vi "List DQMH.vi"() -> ()   [LabVIEW 2020]
uses:
  <vilib>/National Instruments/Tree Map/Tree Map Data.ctl
  Scripting/Event types--enum.ctl
  <vilib>/National Instruments/Tree Map/API/List Roots.vi
  <vilib>/National Instruments/Tree Map/Utility/Into Tree Control Items.vi
  Scripting/DQMH_API.lvlib
  <vilib>/National Instruments/Tree Map/Tree Map.lvlib
  <vilib>/ProgressBar/Progress Bar Dialog.lvclass
panel:
  out "Module":string
  in  "Refresh":bool
  in  "Lists":string(tree) caption="Tree 2"
  in  "Module ID":i32 caption="Numeric"
  out "Running?":bool
  in  "Open API Tester":bool
  in  "Run Request VI":bool
  in  "Show Block Diagram":bool
  in  "Hide Front Panel":bool
  in  "Show Front Panel":bool
  in  "Stop All":bool
  in  "Stop Module":bool
  out "Connector pane":picture
  out "Vi Documentation":string
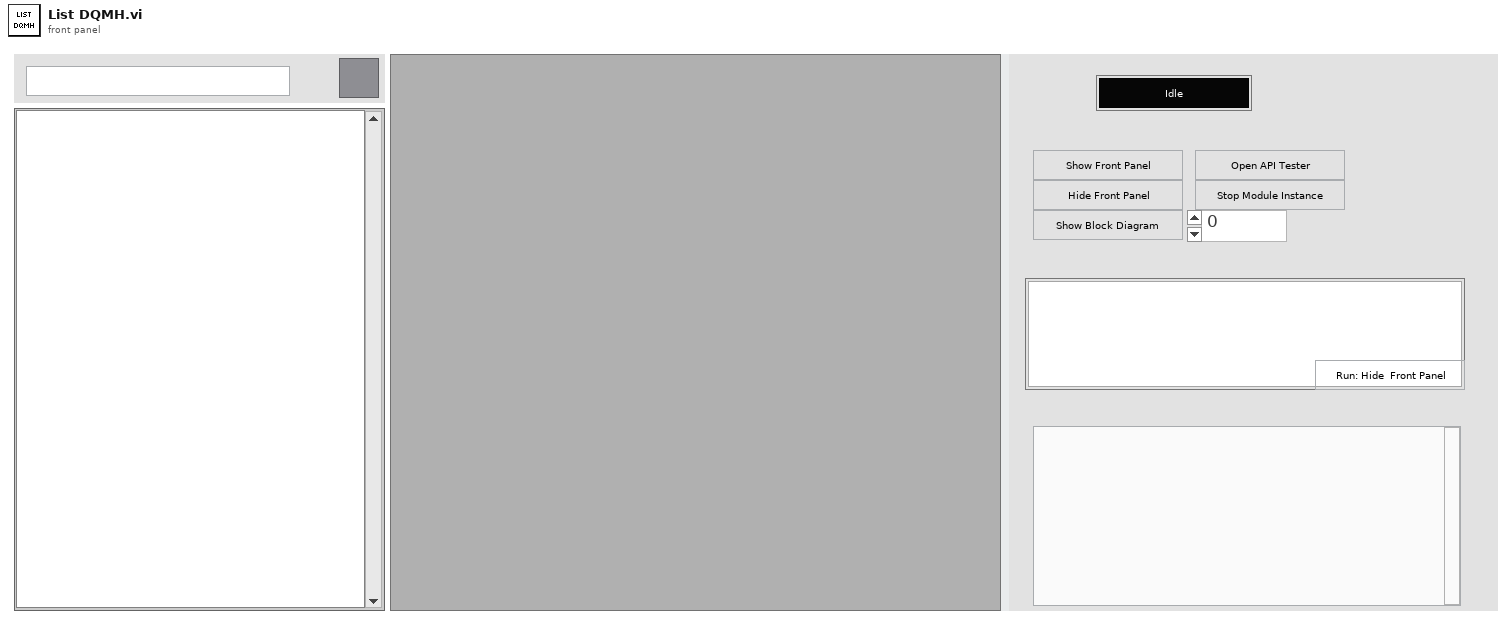
[diagram p1: front panel]
types:
  T1 = enum32{"Invalid", "Standard", "Closed", "Hidden", "Minimized", "Maximized"}
  T2 = enum32{"invalid app kind", "Development System", "Run Time System", "Student Edition", "Embedded LabVIEW", "Evaluation", "Custom"}
  T3 = typedef "Tree Map.lvlib/Tree Map Data.ctl" = map{string, cluster{"Child Paths Set":set{string}, "Name":string, "Data":string, "Attributes":map{string, string}}}
  T4 = cluster{"Core":cluster{"Current VI Reference":refnum<vi>, "Close Panel on Exit?":bool}, "Lists ref":refnum<vi>, "Sub Panel":refnum<vi>, "Tree Map":T3, "References Map":map{string, refnum<vi>}, "vi Ref":refnum<vi>, "Module ID":i32}
  T5 = cluster{"Child Paths Set":set{string}, "Name":string, "Data":string, "Attributes":map{string, string}}
  T6 = cluster{"Current VI Reference":refnum<vi>, "Close Panel on Exit?":bool}
  T7 = typedef "DQMH_API.lvlib/Event types--enum.ctl" = enum16{"Request", "Request and Wait for Reply", "Broadcast"}
  T8 = cluster{"Left Cell String":string, "Child Text":string[], "Child Tag":string, "Item Indent":i32, "Child Only?":bool, "Glyph Index":i32}[]
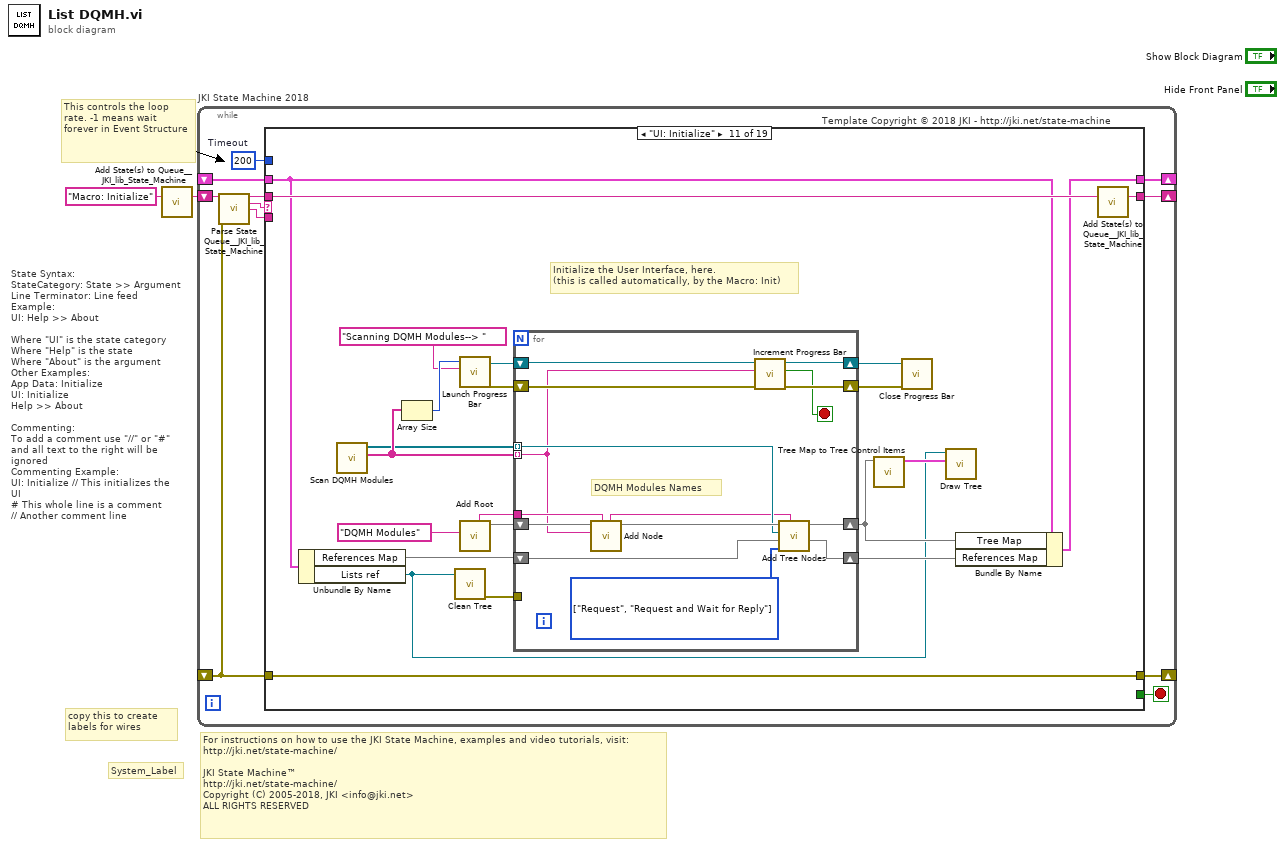
[diagram p0: block diagram]
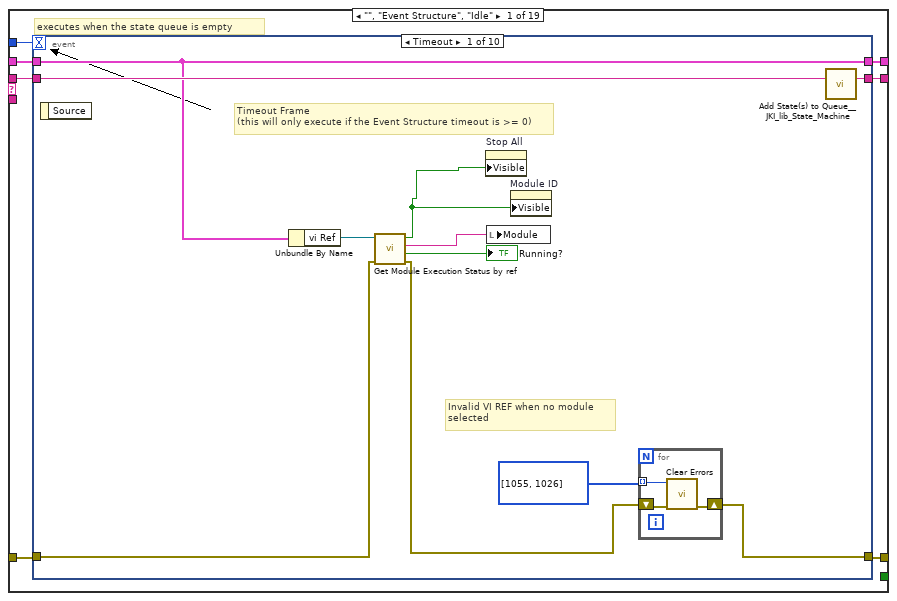
[diagram p2: hidden frame]
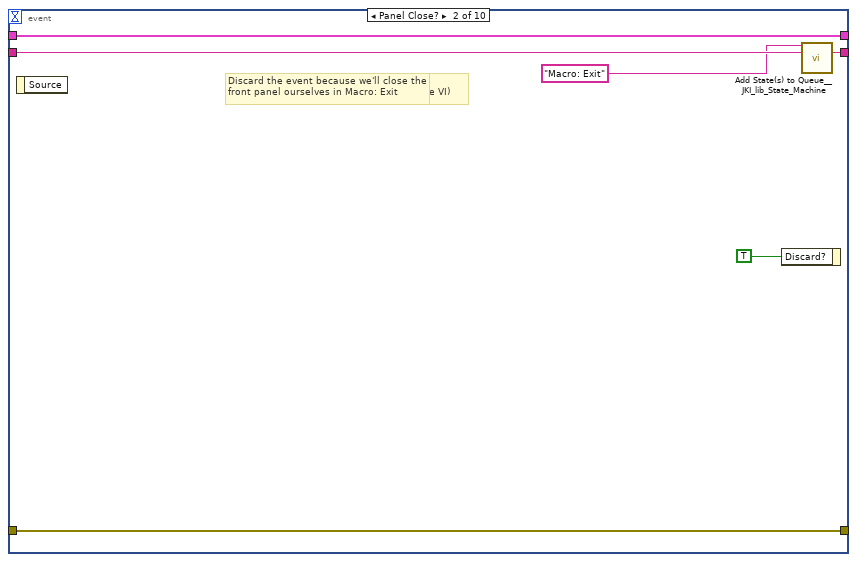
[diagram p3: hidden frame]
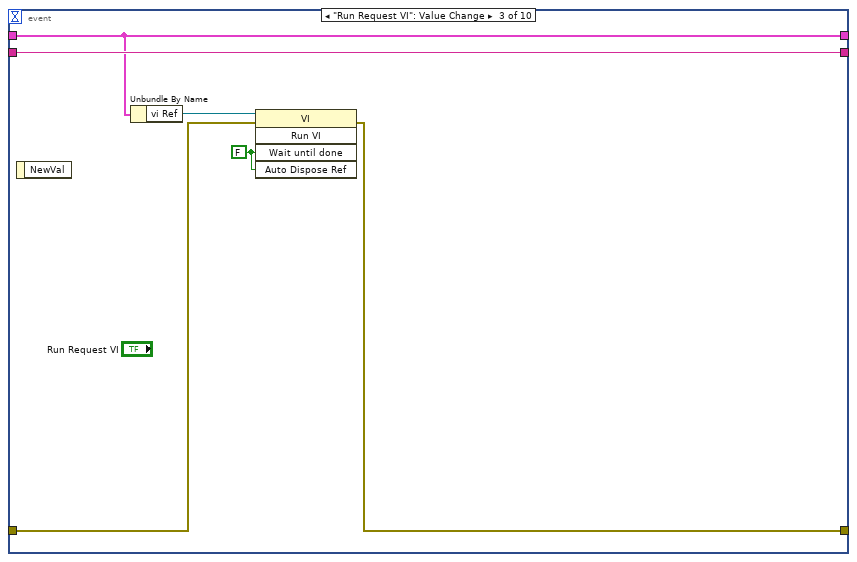
[diagram p4: hidden frame]
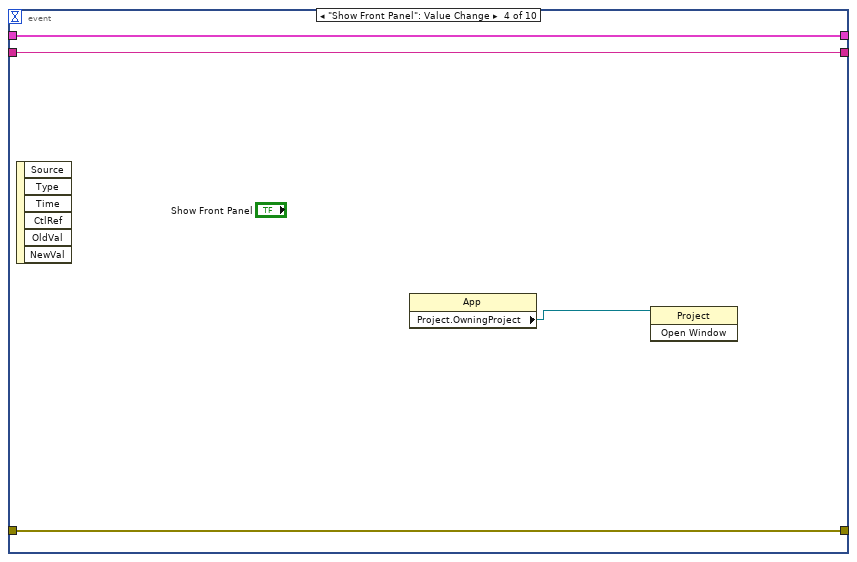
[diagram p5: hidden frame]
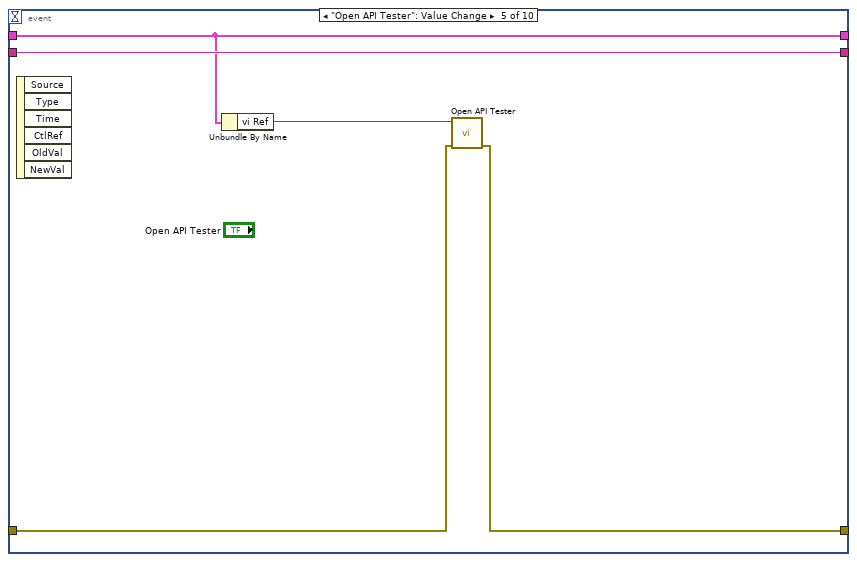
[diagram p6: hidden frame]
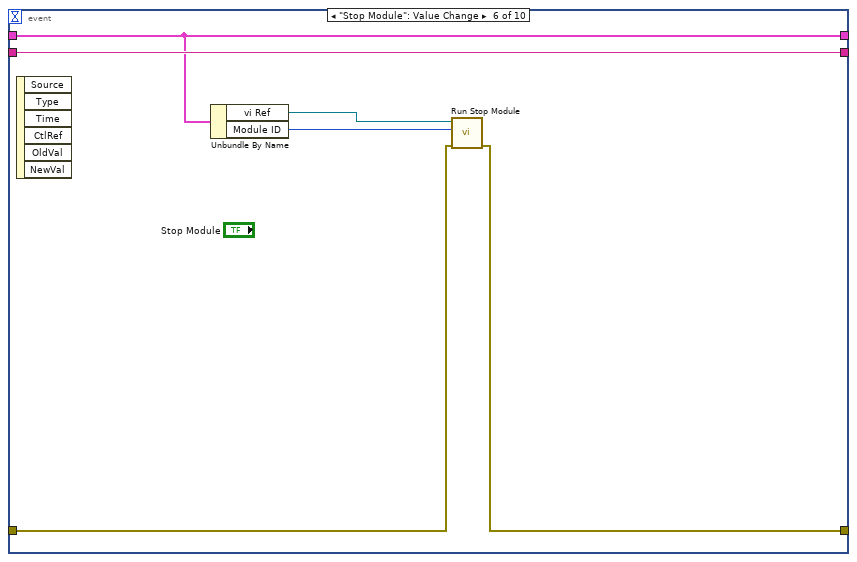
[diagram p7: hidden frame]
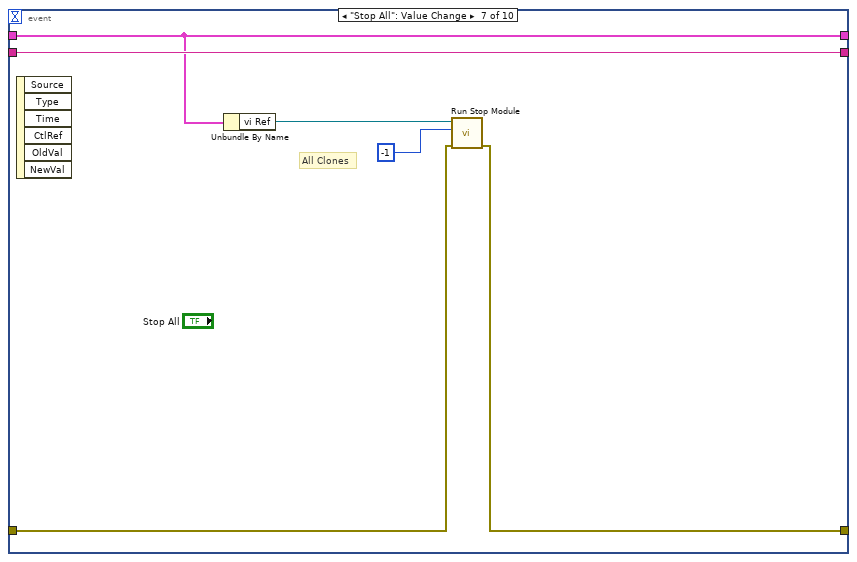
[diagram p8: hidden frame]
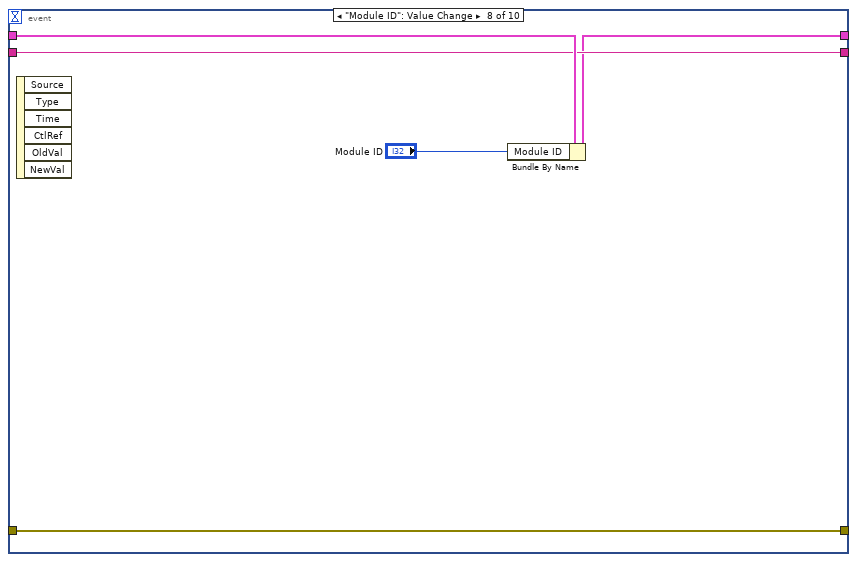
[diagram p9: hidden frame]
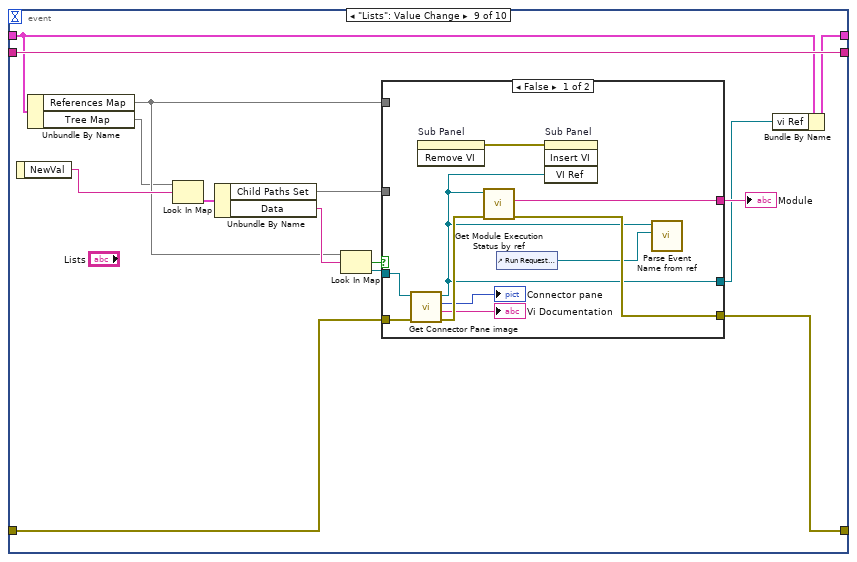
[diagram p10: hidden frame]
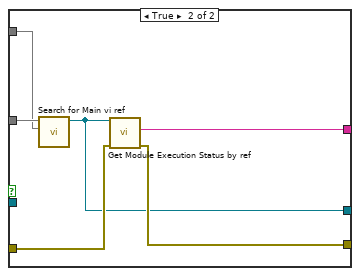
[diagram p11: hidden frame]
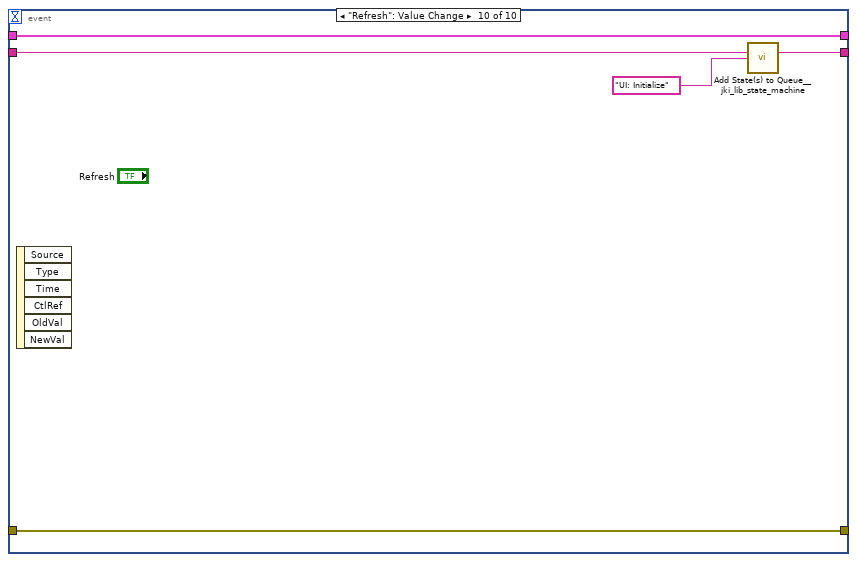
[diagram p12: hidden frame]
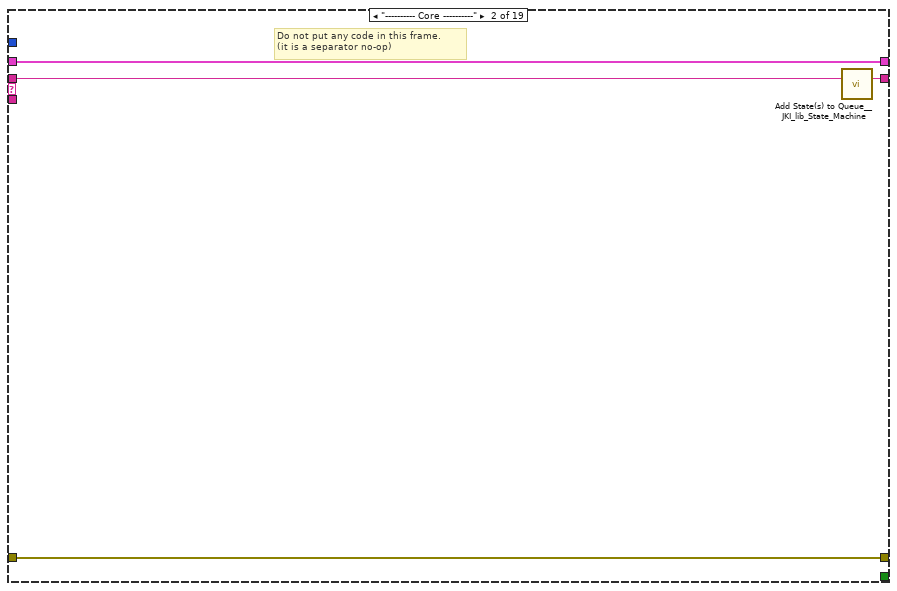
[diagram p13: hidden frame]
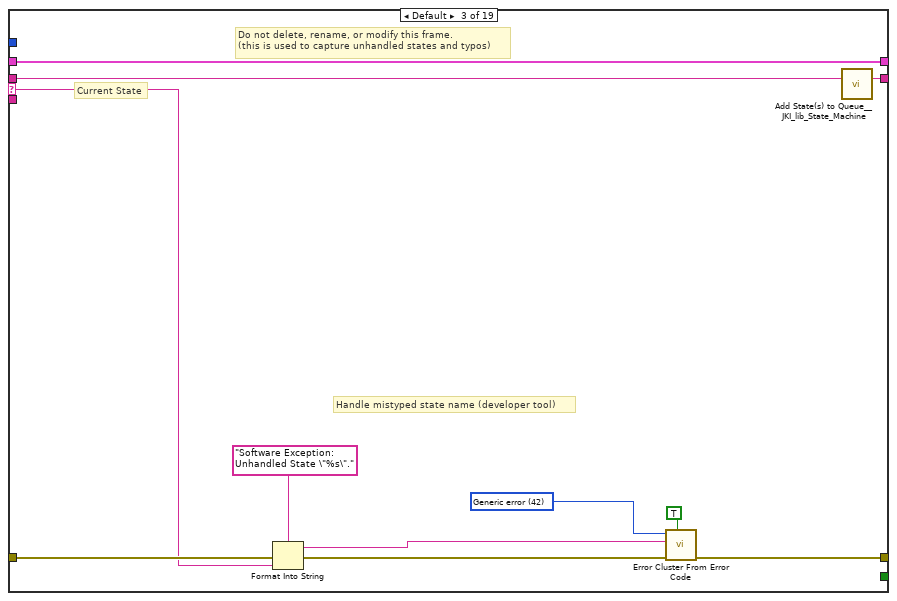
[diagram p14: hidden frame]
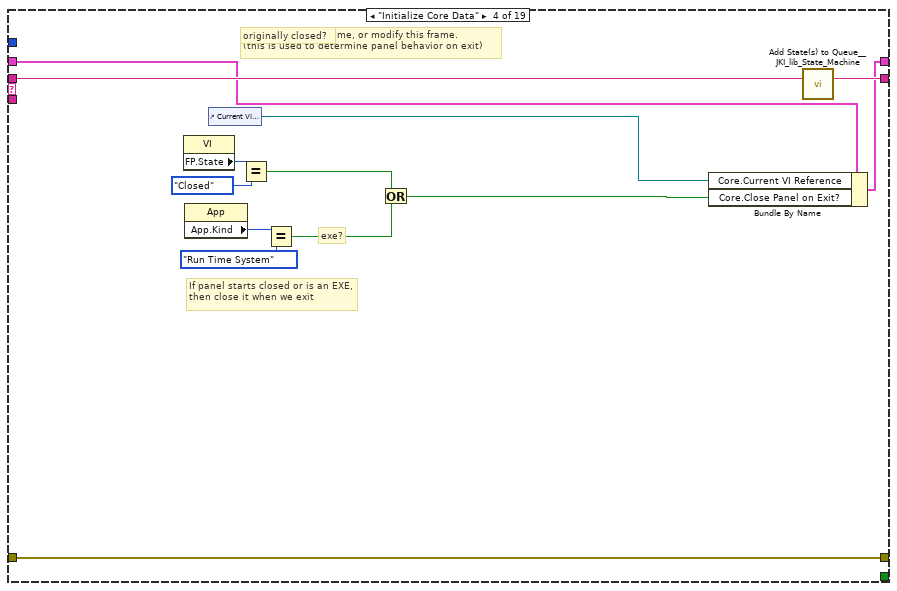
[diagram p15: hidden frame]
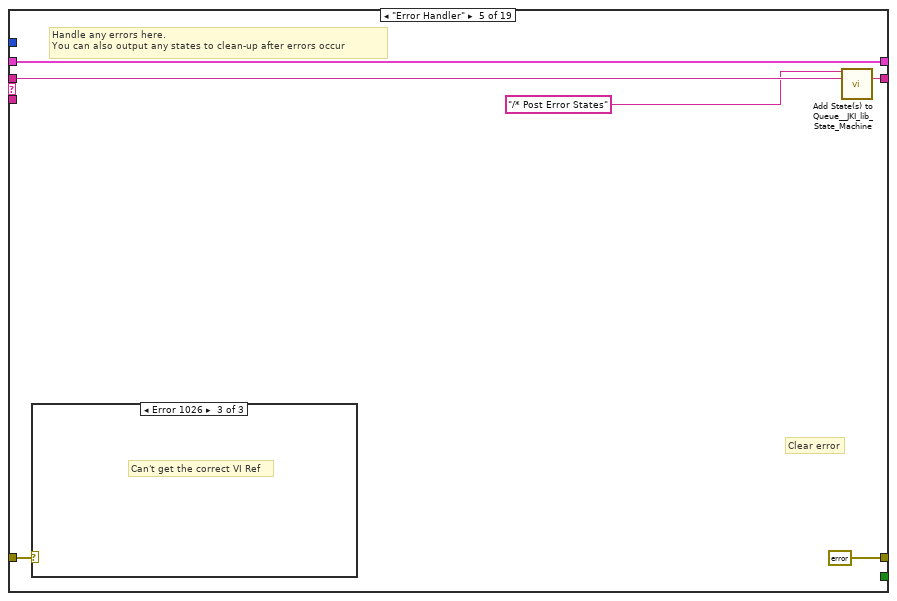
[diagram p16: hidden frame]
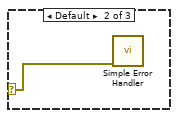
[diagram p18: hidden frame]
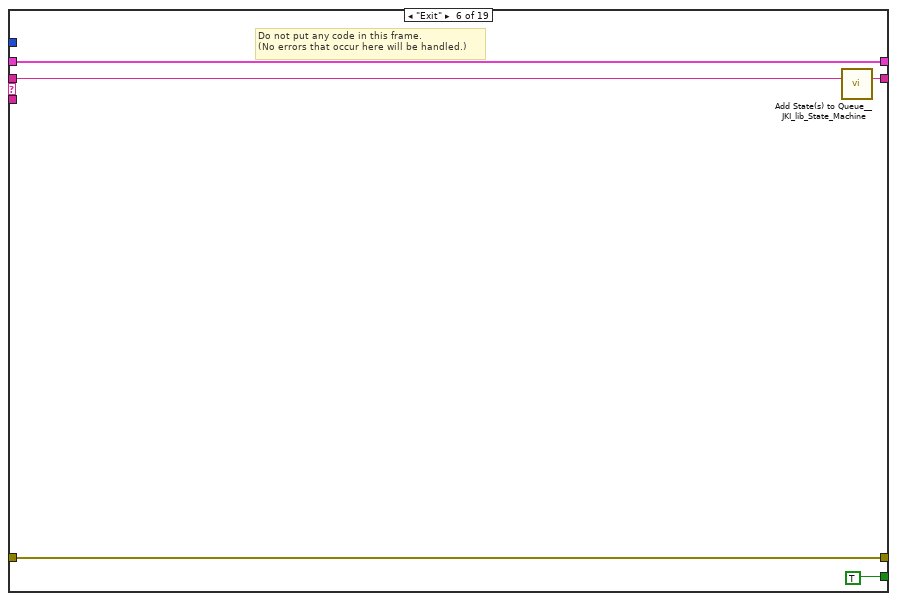
[diagram p19: hidden frame]
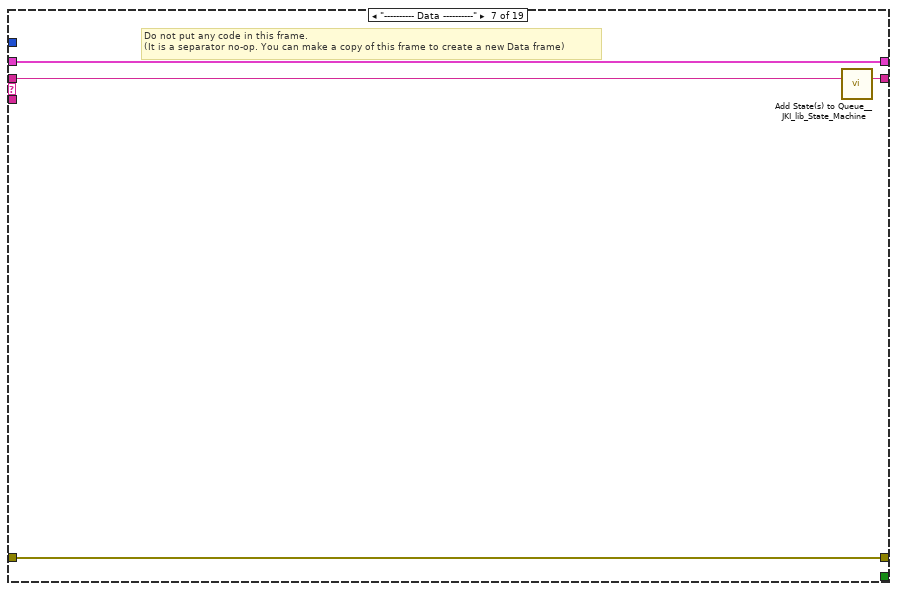
[diagram p20: hidden frame]
diagram:
  # "For instructions on how to use the JKI State Machine, examples and video tutorials, visit:\nhttp://jki.net/state-machine/\n\nJKI State Machine™\nhttp://jki.net/state-machine/\nCopyright (C) 2005-2018, JKI <info@jki.net>\nALL RIGHTS RESERVED"
  # "State Syntax:\nStateCategory: State >> Argument\nLine Terminator: Line feed\nExample:\nUI: Help >> About\n\nWhere \"UI\" is the state category\nWhere \"Help\" is the state\nWhere \"About\" is the argument\nOther Examples:\nApp Data: Initialize\nUI: Initialize\nHelp >> About\n\nCommenting:\nTo add a comment use \"//\" or \"#\" and all text to the right will be ignored\nCommenting Example:\nUI: Initialize // This initializes the UI\n# This whole line is a comment\n// Another comment line"
  # "copy this to create labels for wires"
  # "This controls the loop rate. -1 means wait forever in Event Structure"
  # "System_Label"
  n1 = call <vilib>:"Add State(s) to Queue__JKI_lib_State_Machine.vi"("State(s) in (\"\")"="Macro: Initialize") -> ("States Out"=w2:string)  [unwired: 14 in]
  n2 = while "JKI State Machine 2018" {
    shift-right: [w5] -> _
    shift-left: _ -> [w4]
    shift-right: [w13] -> _
    shift-left: _ -> [w12]
    shift-right: [w7] -> _
    shift-left: w2 -> [w8]
    stop <- w6 stop-if-true
    w3 = 200  # Timeout
    # "Template Copyright © 2018 JKI - http://jki.net/state-machine"
    n3 = call <vilib>:"Parse State Queue__JKI_lib_State_Machine.vi"("State Queue"=w8, "Error In (no error)"=w12) -> ("Remaining States"=w10:string, "Current State"=w11:string, "Arguments"=w9:string)  [unwired: 11 in]
    n4 = case shown="\"UI: Initialize\"" w11 {
      selector: w11 -> [_ _ w113 _ _ _ _ _ _ _ _ _ _ _ _ _ _ _ _]
      tunnel: w10 -> [w18 w111 w117 w135 w140 w147 w151 w162 w170 w179 w198 w221 w232 w297 w302 w312 w316 w320 w324]
      tunnel: w9 -> [_ _ _ _ _ _ _ _ _ _ _ w218 w229 _ _ _ _ _ _]
      tunnel: w4 -> [w16 w109 w115 w124 w138 w144 w149 _ w165 w177 w183 w219 w228 w295 w300 w305 w314 w318 w322]
      tunnel: [w20 w112 w122 w136 errorcluster {"status"=FALSE, "code"=0, "source"=""} ("error out") w148 w152 w163 w174 w180 w202 w222 w233 w298 w303 w313 w317 w321 w325] -> w13
      tunnel: w12 -> [w19 w112 w121 w136 w141 w148 w152 w163 w176 w180 w202 w223 w234 w298 w303 w313 w317 w321 w325]
      tunnel: [w17 w110 w116 w134 w139 w146 w150 w161 w169 w178 w197 w220 w231 w296 w301 w311 w315 w319 w323] -> w7
      tunnel: [_ _ _ _ _ TRUE _ _ _ _ _ _ _ _ _ _ _ _ _] -> w6
      tunnel: [w14 w109 w115 w125 w138 w144 w149 w154 w165 w177 w184 w219 w228 w295 w300 w305 w314 w318 w322] -> w5
      tunnel: w3 -> [w15 _ _ _ _ _ _ _ _ _ _ _ _ _ _ _ _ _ _]
      frame "", "Event Structure", "Idle" {
        # "executes when the state queue is empty"
        n5 = event shown="[0] Timeout" {
          selector: _ -> [_ _ _ _ _ _ _ _ _ _]
          dyn-events: _ -> [_ _ _ _ _ _ _ _ _ _]
          timeout: w15 -> [_ _ _ _ _ _ _ _ _ _]
          tunnel: w18 -> [w28 w39 w44 w49 w53 w59 w65 w70 w79 w105]
          tunnel: [w27 w38 w44 w49 w53 w59 w65 w70 w79 w106] -> w17
          tunnel: w16 -> [w26 w35 w42 w48 w52 w58 w64 w71 w75 w107]
          tunnel: [w29 w40 w45 w50 w55 w61 w67 w72 w86 w108] -> w20
          tunnel: w19 -> [w31 w40 w46 w50 w54 w60 w66 w72 w87 w108]
          tunnel: [w26 w35 w42 w48 w52 w58 w64 w69 w78 w107] -> w14
          event Timeout {
            # "Invalid VI REF when no module \nselected"
            # "Timeout Frame\n(this will only execute if the Event Structure timeout is >= 0)"
            n6 = event-data() -> ()  [unwired: 1 in, 1 out]
            n7 = Unbundle By Name(w26) -> ("vi Ref"=w25:refnum<vi>)
            n8 = call "Get Module Execution Status by ref.vi"("error in"=w31, "Vi Ref"=w25) -> ("error out"=w30:errorcluster, "Running?"=→"Running?":bool, "Module Name"=w24:string, "Is Cloneable"=w21:bool)  [unwired: 6 in]
            n9 = property on="Stop All" class="Bool"("Visible"=w21) -> ()  [unwired: 2 in, 2 out]
            n10 = local write "Module"(w24) -> ()
            n11 = property on="Module ID" class="DigNum (strict)"("Visible"=w21) -> ()  [unwired: 2 in, 2 out]
            n12 = for {
              tunnel: i32[] [1055, 1026] ("specific error code to clear (0: all)") -> [w32] mode=indexing
              shift-right: [w33] -> w29
              shift-left: w30 -> [w34]
              n13 = call <vilib>:"Clear Errors.vi"("error in (no error)"=w34, "specific error code to clear (0: all)"=w32) -> ("error out"=w33:errorcluster)  [unwired: 4 in, 1 out]
            }
            n14 = call <vilib>:"Add State(s) to Queue__JKI_lib_State_Machine.vi"("State(s) in (\"\")"=w28) -> ("States Out"=w27:string)  [unwired: 14 in]
          }
          event Panel Close? {
            # "Discard the event because we'll close the front panel ourselves in Macro: Exit"
            # "Close Panel button (pressed) Event\n(this executes Macro: Exit to terminate the VI)"
            n15 = event-data() -> ()  [unwired: 1 in, 1 out]
            n16 = event-data("Discard?"=TRUE) -> ()  [unwired: 1 in, 1 out]
            n17 = call <vilib>:"Add State(s) to Queue__JKI_lib_State_Machine.vi"("State(s) in Front (\"\")"="Macro: Exit", "State(s) in (\"\")"=w39) -> ("States Out"=w38:string)  [unwired: 13 in]
          }
          event "Run Request VI": Value Change {
            w43 = FALSE ("Wait Until Done")
            n18 = event-data() -> ()  [unwired: 1 in, 1 out]
            n19 = Unbundle By Name(w42) -> ("vi Ref"=w41:refnum<vi>)
            n20 = invoke class="VI" method="Run VI"(reference=w41, error in=w46, "Wait until done"=w43, "Auto Dispose Ref"=w43) -> (error out=w45:errorcluster)  [unwired: 1 in, 4 out]
          }
          event "Show Front Panel": Value Change {
            n21 = event-data() -> ()  [unwired: 1 in, 6 out]
            n22 = property class="App"() -> ("Project.OwningProject"=w47:refnum<vi>)  [unwired: 2 in, 2 out]
            n23 = invoke class="Project" method="Open Window"(reference=w47) -> ()  [unwired: 2 in, 3 out]
          }
          event "Open API Tester": Value Change {
            n24 = event-data() -> ()  [unwired: 1 in, 6 out]
            n25 = Unbundle By Name(w52) -> ("vi Ref"=w51:refnum<vi>)
            n26 = call "Open API Tester.vi"("error in"=w54, "Event vi Ref"=w51) -> ("error out"=w55:errorcluster)  [unwired: 9 in]
          }
          event "Stop Module": Value Change {
            n27 = event-data() -> ()  [unwired: 1 in, 6 out]
            n28 = Unbundle By Name(w58) -> ("vi Ref"=w57:refnum<vi>, "Module ID"=w56:i32)
            n29 = call "Run Stop Module.vi"("error in"=w60, "Module ID"=w56, "Event vi Ref"=w57) -> ("error out"=w61:errorcluster)  [unwired: 8 in]
          }
          event "Stop All": Value Change {
            # "All Clones"
            n30 = event-data() -> ()  [unwired: 1 in, 6 out]
            n31 = Unbundle By Name(w64) -> ("vi Ref"=w63:refnum<vi>)
            n32 = call "Run Stop Module.vi"("error in"=w66, "Module ID"=-1, "Event vi Ref"=w63) -> ("error out"=w67:errorcluster)  [unwired: 8 in]
          }
          event "Module ID": Value Change {
            n33 = event-data() -> ()  [unwired: 1 in, 6 out]
            n34 = Bundle By Name(cluster=w71, "Module ID"="Module ID") -> (w69:T4)
          }
          event "Lists": Value Change {
            n35 = event-data() -> ("NewVal"=w84:string)  [unwired: 1 in]
            n36 = Unbundle By Name(w75) -> ("References Map"=w74:map{string, refnum<vi>}, "Tree Map"=w73:T3)
            n37 = Look In Map(map=w73, key=w84) -> (value=w85:T5)  [unwired: 1 in, 1 out]
            n38 = Unbundle By Name(w85) -> ("Child Paths Set"=w81:set{string}, "Data"=w83:string)
            n39 = Look In Map(map=w74, key=w83) -> (key not found?=w82:bool, value=w76:refnum<vi>)  [unwired: 1 in]
            n40 = case shown="False" w82 {
              tunnel: [w88 w99] -> w77
              tunnel: [w92 w100] -> w80
              tunnel: w74 -> [_ w98]
              tunnel: w81 -> [_ w101]
              tunnel: w76 -> [w91 _]
              tunnel: w87 -> [w96 w103]
              tunnel: [w94 w102] -> w86
              frame False {
                n41 = call "Get Connector Pane image.vi"("error in"=w96, "VI in"=w91) -> ("error out"=w95:errorcluster, "VI Description"=→"Vi Documentation":string, "Connector pane Image"=→"Connector pane":picture, "Vi out"=w88:refnum<vi>)  [unwired: 6 in]
                n42 = invoke on="Sub Panel" class="SubPnl" method="Remove VI"() -> (error out=w97:errorcluster)  [unwired: 3 in, 2 out]
                n43 = call "Get Module Execution Status by ref.vi"("error in"=w95, "Vi Ref"=w88) -> ("error out"=w94:errorcluster, "Module Name"=w92:string)  [unwired: 6 in, 2 out]
                n44 = control-ref of="Run Request VI"() -> (w89:refnum<vi>)
                n45 = invoke on="Sub Panel" class="SubPnl" method="Insert VI"(error in=w97, "VI Ref"=w88) -> ()  [unwired: 2 in, 4 out]
                n46 = call "Parse Event Name from ref.vi"("Boolean Run Request VI"=w89, "VI in"=w88) -> ()  [unwired: 10 in]
              }
              frame True {
                n47 = call "Search for Main vi ref.vi"("map"=w98, "Child Paths Set"=w101) -> ("Main vi Ref"=w99:refnum<vi>)  [unwired: 9 in]
                n48 = call "Get Module Execution Status by ref.vi"("error in"=w103, "Vi Ref"=w99) -> ("error out"=w102:errorcluster, "Module Name"=w100:string)  [unwired: 6 in, 2 out]
              }
            }
            "Module" <- w80
            n49 = Bundle By Name(cluster=w75, "vi Ref"=w77) -> (w78:T4)
          }
          event "Refresh": Value Change {
            n50 = event-data() -> ()  [unwired: 1 in, 6 out]
            n51 = call <vilib>:"Add State(s) to Queue__jki_lib_state_machine.vi"("State(s) in (\"\")"=w105, "State(s) at Back (\"\")"="UI: Initialize" ("State(s) at Back (\"\")")) -> ("States Out"=w106:string)  [unwired: 13 in]
          }
        }
      }
      frame "---------- Core ----------" {
        # "Do not put any code in this frame.\n(it is a separator no-op)"
        n52 = call <vilib>:"Add State(s) to Queue__JKI_lib_State_Machine.vi"("State(s) in (\"\")"=w111) -> ("States Out"=w110:string)  [unwired: 14 in]
      }
      frame Default {
        w119 = 42 items=["No error", "Argument error", "Memory is full", "Out of zone", "End of file", "File already open", "Generic file I/O error", "File not found", "File permission error", "Disk is full", "Duplicate path", "Too many files open", "System feature not enabled", "Resource file not found", "Cannot add resource", "Resource not found", "Image not found", "Image memory error", "Pen does not exist", "Config type invalid", "Config token not found", "Config parse error", "Config memory error", "Bad external code format", "Bad external code offset", "External code not present", "Null window", "Destroy window error", "Null menu", "Print aborted", "Bad print record", "Print driver error", "Windows error during printing", "Memory error during printing", "Print dialog error", "Generic print error", "Invalid device refnum", "Device not found", "Device parameter error", "Device unit error", "Cannot open device", "Device call aborted", "Generic error", "Cancelled by user", "Object ID too low", "Object ID too high", "Object not in heap", "Unknown heap", "Unknown object (invalid DefProc)", "Unknown object (DefProc not in table)", "Message out of range", "Invalid (null) method", "Unknown message", "Manager call not supported", "Bad address", "Network operation in progress", "Network operation timed out", "Connection is busy", "Network attribute not supported", "Network error", "Address in use", "System out of memory", "Connection aborted", "Connection refused", "Not connected", "Already connected", "Connection closed", "Initialization error (interapplication manager)", "Bad occurrence", "Wait on unbound occurrence handler", "Occurrence queue overflow", "Datalog type conflict", "Unused", "Unrecognized type (interapplication manager)", "Memory corrupt", "Failed to make temporary DLL", "Old CIN version", "Drag socket not found", "Failed to load drop-object", "Failed to register OLE object", "Failed to release OLE object", "Format specifier type mismatch", "Unknown format specifier", "Too few format specifiers", "Too many format specifiers", "Scan failed", "Newer CIN version", "Error converting to variant", "Runtime menu error", "Password tampered", "Variant attribute not found", "Incompatible variant data type", "Event data is not available", "Event Store is not present", "Occurrence is not found", "Event Queue is not created", "Event info is not available", "Refnum passed is NULL", "Error retrieving Class GUID", "Error retrieving CoClass GUID", "Error retrieving TypeLib GUID.", "Bad built application magic bytes.", "Specific driver is different from the specific driver associated with the Logical Name.", "There is no session opened to the class driver.", "Max Error", "MAX - Error with config objects", "MAX - Error loading configuration", "MAX - Group not supported"]
        # "Current State"
        # "Do not delete, rename, or modify this frame.\n(this is used to capture unhandled states and typos)"
        # "Handle mistyped state name (developer tool)"
        n53 = Format Into String(format string="Software Exception: Unhandled State \"%s\"." ("message"), error in=w121, w113) -> (resulting string=w118:string, error out=w123:errorcluster)  [unwired: 1 in]
        n54 = call <vilib>:"Error Cluster From Error Code.vi"("show call chain? (False)"=TRUE, "error in (no error)"=w123, "error message (\"\")"=w118, "error code (0)"=w119) -> ("error out"=w122:errorcluster)  [unwired: 5 in]
        n55 = call <vilib>:"Add State(s) to Queue__JKI_lib_State_Machine.vi"("State(s) in (\"\")"=w117) -> ("States Out"=w116:string)  [unwired: 14 in]
      }
      frame "Initialize Core Data" {
        # "Do not delete, rename, or modify this frame.\n(this is used to determine panel behavior on exit)"
        # "originally closed?"
        # "exe?"
        # "If panel starts closed or is an EXE, then close it when we exit"
        n56 = property class="VI"() -> ("FP.State"=w128:T1)  [unwired: 2 in, 2 out]
        n57 = property class="App"() -> ("App.Kind"=w133:T2)  [unwired: 2 in, 2 out]
        n58 = control-ref of="Current VI Reference"() -> (w129:refnum<vi>)
        n59 = Equal?(x=w128, y=T1."Closed" ("Front Panel Window:State")) -> (x = y?=w126:bool)
        n60 = Equal?(x=w133, y=T2."Run Time System" ("Application:Kind")) -> (x = y?=w131:bool)
        n61 = Or(x=w126, y=w131) -> (x .or. y?=w130:bool)
        n62 = Bundle By Name(cluster=w124, "Core.Current VI Reference"=w129, "Core.Close Panel on Exit?"=w130) -> (w125:T4)
        n63 = call <vilib>:"Add State(s) to Queue__JKI_lib_State_Machine.vi"("State(s) in (\"\")"=w135) -> ("States Out"=w134:string)  [unwired: 14 in]
      }
      frame "Error Handler" {
        # "Handle any errors here.\nYou can also output any states to clean-up after errors occur"
        # "Clear error"
        n64 = case shown="Error 1026" w141 {
          selector: w141 -> [_ w143 _]
          frame No Error {
          }
          frame Default {
            n65 = call <vilib>:"Simple Error Handler.vi"("error in (no error)"=w143) -> ()  [unwired: 4 in, 5 out]
          }
          frame Error {
            # "Can't get the correct VI Ref"
          }
        }
        n66 = call <vilib>:"Add State(s) to Queue__JKI_lib_State_Machine.vi"("State(s) in Front (\"\")"="/* Post Error States", "State(s) in (\"\")"=w140) -> ("States Out"=w139:string)  [unwired: 13 in]
      }
      frame "Exit" {
        # "Do not put any code in this frame.\n(No errors that occur here will be handled.)"
        n67 = call <vilib>:"Add State(s) to Queue__JKI_lib_State_Machine.vi"("State(s) in (\"\")"=w147) -> ("States Out"=w146:string)  [unwired: 14 in]
      }
      frame "---------- Data ----------" {
        # "Do not put any code in this frame.\n(It is a separator no-op. You can make a copy of this frame to create a new Data frame)"
        n68 = call <vilib>:"Add State(s) to Queue__JKI_lib_State_Machine.vi"("State(s) in (\"\")"=w151) -> ("States Out"=w150:string)  [unwired: 14 in]
      }
      frame "Data: Initialize" {
        w153 = -1  # Module ID
        w155 = refnum<vi> refnum  # vi Ref
        w156 = map{string, refnum<vi>} {}  # References Map
        w157 = T3 {}  # Tree Map
        w160 = T6 {"Current VI Reference"=refnum, "Close Panel on Exit?"=FALSE}  # Core
        # "Data names and types of shift register data are defined by this bundle."
        # "Initialize the shift-register data, here.\n(data names are defined by what you wire into the bundle function)"
        n69 = control-ref of="Lists ref"() -> (w159:refnum<vi>)
        n70 = control-ref of="Sub Panel"() -> (w158:refnum<vi>)
        n71 = Bundle("Core"=w160, "Lists ref"=w159, "Sub Panel"=w158, "Tree Map"=w157, "References Map"=w156, "vi Ref"=w155, "Module ID"=w153) -> (w154:T4)  [unwired: 1 in]
        n72 = call <vilib>:"Add State(s) to Queue__JKI_lib_State_Machine.vi"("State(s) in (\"\")"=w162) -> ("States Out"=w161:string)  [unwired: 14 in]
      }
      frame "Data: Cleanup" {
        # "Cleanup any data and references, here.\n(this is called automatically, by the Macro: Exit)"
        n73 = Unbundle By Name(w165) -> ("Lists ref"=w166:refnum<vi>, "References Map"=w168:map{string, refnum<vi>}, "vi Ref"=w167:refnum<vi>, "Core.Current VI Reference"=w164:refnum<vi>)
        n74 = Close Reference(reference=w164, error in (no error)=w176) -> (error out=w175:errorcluster)
        n75 = Close Reference(reference=w167) -> (error out=w173:errorcluster)  [unwired: 1 in]
        n76 = call "Close vi references.vi"("map"=w168) -> ("error out"=w172:errorcluster)  [unwired: 10 in]
        n77 = call "Clean Tree.vi"("TreeControl in"=w166) -> ("error out"=w171:errorcluster)  [unwired: 10 in]
        n78 = Merge Errors(w171, w172, w173, w175) -> (w174:errorcluster)
        n79 = call <vilib>:"Add State(s) to Queue__JKI_lib_State_Machine.vi"("State(s) in (\"\")"=w170) -> ("States Out"=w169:string)  [unwired: 14 in]
      }
      frame "---------- UI ----------" {
        # "Do not put any code in this frame.\n(It is a separator no-op. You can make a copy of this frame to create a new UI frame)"
        n80 = call <vilib>:"Add State(s) to Queue__JKI_lib_State_Machine.vi"("State(s) in (\"\")"=w179) -> ("States Out"=w178:string)  [unwired: 14 in]
      }
      frame "UI: Initialize" {
        # "Initialize the User Interface, here.\n(this is called automatically, by the Macro: Init)"
        n81 = Unbundle By Name(w183) -> ("References Map"=w182:map{string, refnum<vi>}, "Lists ref"=w181:refnum<vi>)
        n82 = call "Scan DQMH Modules.vi"() -> ("Modules List"=w196:string[], "DQMH Modules"=w192:refnum<vi>[])  [unwired: 8 in, 2 out]
        n83 = Array Size(array=w196) -> (size(s)=w195:i32)
        n84 = call "Clean Tree.vi"("TreeControl in"=w181) -> ("error out"=w199:errorcluster)  [unwired: 10 in]
        n85 = call <vilib>:"Launch Progress Bar.vi"("Main Title (\"Working...\")"="Scanning DQMH Modules--> " ("Main Title (\"Working...\")"), "Total Count"=w195) -> ("error out"=w201:errorcluster, "Progress Bar Dialog"=w193:refnum<class "Progress Bar Dialog.lvclass">)  [unwired: 8 in]
        n86 = call <vilib>:"Add Root.vi"("New Root Name"="DQMH Modules") -> ("Tree Map Out"=w189:T3, "Root Path"=w190:string)  [unwired: 9 in]
        n87 = for {
          shift-right: [w210] -> w186
          shift-left: w189 -> [w215]
          tunnel: w196 -> [w203] mode=indexing
          tunnel: w190 -> [w214]
          tunnel: w192 -> [w208] mode=indexing
          shift-right: [w211] -> w185
          shift-left: w182 -> [w212]
          shift-right: [w206] -> w194
          shift-left: w193 -> [w207]
          shift-right: [w217] -> w200
          shift-left: w201 -> [w216]
          tunnel: w199 -> [_]
          stop <- w205 stop-if-true
          w209 = T7[] [enum."Request", enum."Request and Wait for Reply"] items=["Request", "Request and Wait for Reply", "Broadcast"] ("Event Types")
          # "DQMH Modules Names"
          n88 = call <vilib>:"Add Node.vi"("Parent Path"=w214, "New Node Name"=w203, "Tree Map In"=w215) -> ("Tree Map Out"=w213:T3, "New Node Path"=w204:string)  [unwired: 6 in, 1 out]
          n89 = call <vilib>:"Increment Progress Bar.vi"("error in (no error)"=w216, "Step Name (\"\")"=w203, "Progress Bar Dialog in"=w207) -> ("error out"=w217:errorcluster, "Cancelled?"=w205:bool, "Progress Bar Dialog out"=w206:refnum<class "Progress Bar Dialog.lvclass">)  [unwired: 6 in]
          n90 = call "Add Tree Nodes.vi"("Root path"=w204, "Event Types"=w209, "map ref in"=w212, "DQMH Lib In"=w208, "Tree Map in"=w213) -> ("map ref out"=w211:map{string, refnum<vi>}, "Tree Map out"=w210:T3)  [unwired: 5 in]
        }
        n91 = call <vilib>:"Tree Map to Tree Control Items.vi"("Tree Map In"=w186) -> ("Tree Control Items"=w191:T8)  [unwired: 10 in]
        n92 = call <vilib>:"Close Progress Bar.vi"("error in (no error)"=w200, "Progress Bar Dialog"=w194) -> ()  [unwired: 9 in, 1 out]
        n93 = call "Draw Tree.vi"("Tree Control Items"=w191, "TreeControl in"=w181) -> ()  [unwired: 9 in, 1 out]
        n94 = Bundle By Name(cluster=w183, "Tree Map"=w186, "References Map"=w185) -> (w184:T4)
        n95 = call <vilib>:"Add State(s) to Queue__JKI_lib_State_Machine.vi"("State(s) in (\"\")"=w198) -> ("States Out"=w197:string)  [unwired: 14 in]
      }
      frame "UI: Cursor Set" {
        # "Argument"
        # "Set and Unset Cursor Busy.\n(Usage: \"UI: Cursor Set >> Busy|Idle\")"
        n96 = case shown="\"Idle\", Default" w218 {
          tunnel: w223 -> [w225 w227]
          tunnel: [w224 w226] -> w222
          frame "Idle", Default {
            n97 = call <vilib>:"Unset Busy.vi"("error in (no error)"=w225) -> ("error out"=w224:errorcluster)  [unwired: 10 in]
          }
          frame "Busy" {
            n98 = call <vilib>:"Set Busy.vi"("error in (no error)"=w227) -> ("error out"=w226:errorcluster)  [unwired: 9 in, 1 out]
          }
        }
        n99 = call <vilib>:"Add State(s) to Queue__JKI_lib_State_Machine.vi"("State(s) in (\"\")"=w221) -> ("States Out"=w220:string)  [unwired: 14 in]
      }
      frame "UI: Front Panel State" {
        # "Argument"
        # "Set Front Panel Open or Closed\n(Usage: \"UI: Front Panel State >> Open|Close\")"
        n100 = Unbundle By Name(w228) -> ("Core.Current VI Reference"=w230:refnum<vi>)
        n101 = case shown="\"Open\", \"Standard\", Default" w229 {
          tunnel: w234 -> [w240 w253 w264 w276 w288]
          tunnel: [w241 w254 w265 w277 w289] -> w233
          tunnel: w230 -> [_ _ _ _ _]
          frame "Open", "Standard", Default {
            w235 = T1."Standard" ("State")
            n102 = property class="VI"(error in=w240) -> (reference out=w238:refnum<vi>, error out=w239:errorcluster, "FP.State"=w237:T1)  [unwired: 1 in]
            n103 = Not Equal?(x=w237, y=w235) -> (x != y?=w236:bool)
            n104 = case shown="True" w236 {
              tunnel: [w246 w247] -> w241
              tunnel: w239 -> [w245 w247]
              tunnel: w238 -> [w243 _]
              tunnel: w235 -> [w242 _]
              frame True {
                n105 = invoke class="VI" method="FP.Open"(reference=w243, error in=w245, "Activate"=TRUE, "State"=w242) -> (error out=w246:errorcluster)  [unwired: 1 in, 4 out]
              }
              frame False {
              }
            }
          }
          frame "Close", "Closed" {
            n106 = property class="VI"(error in=w253) -> (reference out=w251:refnum<vi>, error out=w252:errorcluster, "FP.State"=w249:T1)  [unwired: 1 in]
            n107 = Not Equal?(x=w249, y=T1."Closed" ("Front Panel Window:State")) -> (x != y?=w248:bool)
            n108 = case shown="True" w248 {
              tunnel: [w255 w258] -> w254
              tunnel: w252 -> [w255 w257]
              tunnel: w251 -> [_ w256]
              frame False {
              }
              frame True {
                n109 = invoke class="VI" method="FP.Close"(reference=w256, error in=w257) -> (error out=w258:errorcluster)  [unwired: 1 in, 2 out]
              }
            }
          }
          frame "Hidden", "Hide" {
            w259 = T1."Hidden" ("State")
            n110 = property class="VI"(error in=w264) -> (reference out=w262:refnum<vi>, error out=w263:errorcluster, "FP.State"=w261:T1)  [unwired: 1 in]
            n111 = Not Equal?(x=w261, y=w259) -> (x != y?=w260:bool)
            n112 = case shown="True" w260 {
              tunnel: [w269 w270] -> w265
              tunnel: w263 -> [w268 w270]
              tunnel: w262 -> [w267 _]
              tunnel: w259 -> [w266 _]
              frame True {
                n113 = invoke class="VI" method="FP.Open"(reference=w267, error in=w268, "State"=w266) -> (error out=w269:errorcluster)  [unwired: 2 in, 4 out]
              }
              frame False {
              }
            }
          }
          frame "Minimize", "Minimized" {
            w271 = T1."Minimized" ("State")
            n114 = property class="VI"(error in=w276) -> (reference out=w274:refnum<vi>, error out=w275:errorcluster, "FP.State"=w273:T1)  [unwired: 1 in]
            n115 = Not Equal?(x=w273, y=w271) -> (x != y?=w272:bool)
            n116 = case shown="True" w272 {
              tunnel: [w281 w282] -> w277
              tunnel: w275 -> [w280 w282]
              tunnel: w274 -> [w279 _]
              tunnel: w271 -> [w278 _]
              frame True {
                n117 = invoke class="VI" method="FP.Open"(reference=w279, error in=w280, "State"=w278) -> (error out=w281:errorcluster)  [unwired: 2 in, 4 out]
              }
              frame False {
              }
            }
          }
          frame "Maximize", "Maximized" {
            w283 = T1."Maximized" ("State")
            n118 = property class="VI"(error in=w288) -> (reference out=w286:refnum<vi>, error out=w287:errorcluster, "FP.State"=w285:T1)  [unwired: 1 in]
            n119 = Not Equal?(x=w285, y=w283) -> (x != y?=w284:bool)
            n120 = case shown="True" w284 {
              tunnel: [w293 w294] -> w289
              tunnel: w287 -> [w292 w294]
              tunnel: w286 -> [w291 _]
              tunnel: w283 -> [w290 _]
              frame True {
                n121 = invoke class="VI" method="FP.Open"(reference=w291, error in=w292, "State"=w290) -> (error out=w293:errorcluster)  [unwired: 2 in, 4 out]
              }
              frame False {
              }
            }
          }
        }
        n122 = call <vilib>:"Add State(s) to Queue__JKI_lib_State_Machine.vi"("State(s) in (\"\")"=w232) -> ("States Out"=w231:string)  [unwired: 14 in]
      }
      frame "---------- Macro ----------" {
        # "Do not put any code in this frame.\n(It is a separator no-op. You can make a copy of this frame to create a new Macro frame)"
        n123 = call <vilib>:"Add State(s) to Queue__JKI_lib_State_Machine.vi"("State(s) in (\"\")"=w297) -> ("States Out"=w296:string)  [unwired: 14 in]
      }
      frame "Macro: Initialize" {
        w299 = "Data: Initialize\nInitialize Core Data\nUI: Initialize\nUI: Front Panel State >> Open"  # Data: Initialize Initialize Core Data UI: Initialize UI: Front Panel State >> Open
        # "Initialization Macro\n(This is called once, when the VI starts)"
        n124 = call <vilib>:"Add State(s) to Queue__JKI_lib_State_Machine.vi"("State(s) in Front (\"\")"=w299, "State(s) in (\"\")"=w302) -> ("States Out"=w301:string)  [unwired: 13 in]
      }
      frame "Macro: Exit" {
        # "Exit Macro\n(This is called once, when the VI exits)"
        n125 = Unbundle By Name(w305) -> ("Core.Close Panel on Exit?"=w304:bool)
        n126 = Select(t="UI: Front Panel State >> Close", s=w304, f="") -> (s? t:f=w308:string)
        n127 = call <vilib>:"Add State(s) to Queue__JKI_lib_State_Machine.vi"("State(s) in (\"\")"=w308, "State(s) at Back (\"\")"="Data: Cleanup\nExit") -> ("States Out"=w306:string)  [unwired: 13 in]
        n128 = call <vilib>:"Add State(s) to Queue__JKI_lib_State_Machine.vi"("State(s) in Front (\"\")"=w306, "State(s) in (\"\")"=w312) -> ("States Out"=w311:string)  [unwired: 13 in]
      }
      frame "---------- New Category ----------" {
        # "Template Separator\n(You can make a copy of, or modify, this frame)"
        n129 = call <vilib>:"Add State(s) to Queue__JKI_lib_State_Machine.vi"("State(s) in (\"\")"=w316) -> ("States Out"=w315:string)  [unwired: 14 in]
      }
      frame "New Category: 1" {
        # "Your code here.\n(You can make a copy of, or modify, this frame)"
        n130 = call <vilib>:"Add State(s) to Queue__JKI_lib_State_Machine.vi"("State(s) in (\"\")"=w320) -> ("States Out"=w319:string)  [unwired: 14 in]
      }
      frame "New Category: 2" {
        # "Your code here.\n(You can make a copy of, or modify, this frame)"
        n131 = call <vilib>:"Add State(s) to Queue__JKI_lib_State_Machine.vi"("State(s) in (\"\")"=w324) -> ("States Out"=w323:string)  [unwired: 14 in]
      }
    }
  }
